vi "MassBandAnalysis.vi"(7 "Settings":T2 {"Bands" items=["No Bands", "", "Test2", "test3", "Test"]; "Smoothing" items=["No smoothing"=0, "1/4 semitone"=25, "1/2 semitone"=50, "1 semitone"=100, "2 semitones"=200]; "View Type" items=["As measured", "Normalize", "Separate", "Complex Average", "Real Average"]}) -> ()   [LabVIEW 2024]
uses:
  ViolinSubs/Mic/Mic_Global.vi
  <vilib>/Analysis/NI_AALBase.lvlib
panel:
  out "Histogram Graph":T1(graph)=[{"X Values"=[17.709212807875016, 17.747951602292737, 17.78669039671046, 17.82542919112818, 17.8641679855459, 17.902906779963622, 17.941645574381344, 17.980384368799065, 18.019123163216786, 18.057861957634508], "Histogram: h(x)"=[2, 0, 0, 0, 0, 0, 1, 1, 0, 1]}, {"X Values"=[12.63540113055175, 12.712222839510153, 12.789044548468555, 12.865866257426957, 12.942687966385359, 13.01950967534376, 13.096331384302163, 13.173153093260565, 13.249974802218967, 13.326796511177369], "Histogram: h(x)"=[1, 0, 0, 1, 1, 0, 0, 1, 0, 1]}, {"X Values"=[19.841497748567125, 19.924216631266706, 20.006935513966287, 20.089654396665868, 20.17237327936545, 20.25509216206503, 20.33781104476461, 20.42052992746419, 20.50324881016377, 20.585967692863353], "Histogram: h(x)"=[1, 0, 1, 0, 0, 0, 0, 1, 0, 2]}, {"X Values"=[13.972825761972334, 14.01058377321214, 14.048341784451946, 14.086099795691752, 14.123857806931557, 14.161615818171363, 14.199373829411169, 14.237131840650974, 14.27488985189078, 14.312647863130586], "Histogram: h(x)"=[1, 0, 1, 1, 0, 0, 0, 1, 0, 1]}]
  in  "intervals":i32=10
  in  "Path":path=path "/Users/crogers/Desktop/Violin/ViolinData/Testing"
  out "# Lines":i32=5
  out "Average FRF":cluster{"x0":dbl, "df":dbl, dbl[]}[](graph)=[{"x0"=0.0, "df"=1.0, array[7000 elements]}, {"x0"=0.0, "df"=1.0, array[7000 elements]}, {"x0"=0.0, "df"=1.0, array[7000 elements]}, {"x0"=0.0, "df"=1.0, array[7000 elements]}, {"x0"=0.0, "df"=1.0, array[7000 elements]}]
  # "1. select the instrument folder (it will get all the TRF files in each test)\n2. hit run\n3. mess with settings (need to do a first run to get the band dropdown \n    to be correct)"
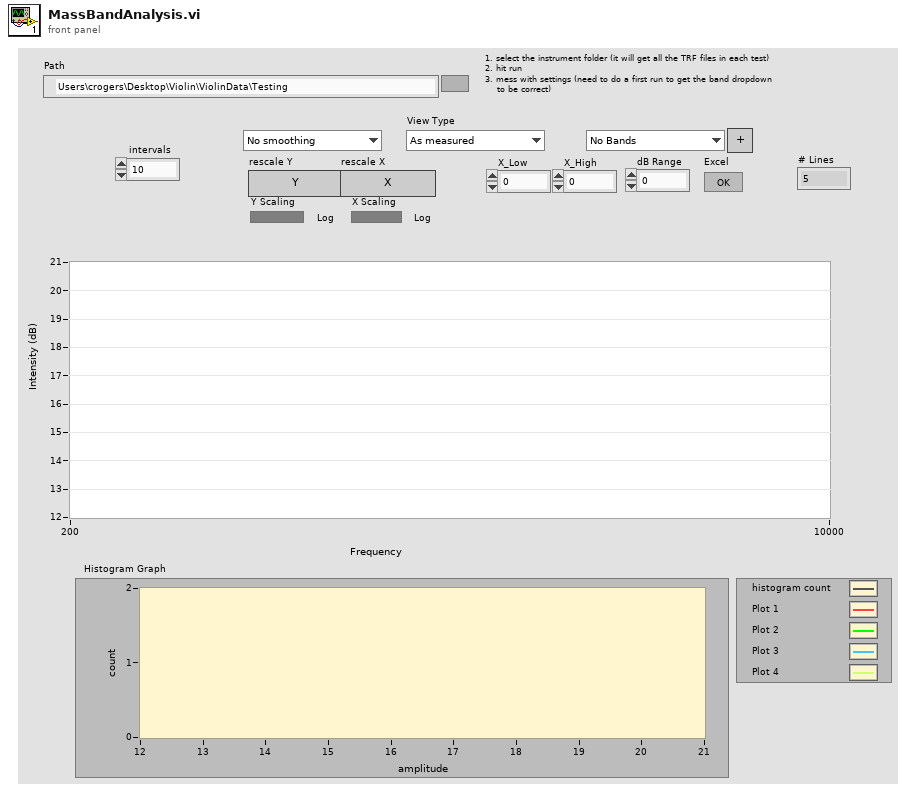
[diagram p1: front panel]
types:
  T1 = cluster{"X Values":dbl[], "Histogram: h(x)":i32[]}[]
  T2 = cluster{"View Type":u16, "Smoothing":u16, "Bands":u16, "New Band":bool, "rescale Y":bool, "rescale X":bool, "X_Low":dbl, "X_High":dbl, "dB Range":dbl, "Excel":bool, "Y Scaling":bool, "X Scaling":bool}
  T3 = cluster{"Start freq":dbl, "Hz resolution":dbl, cdb[]}
  T4 = cluster{"Alerts":bool, "Log X Axis":bool, "dB scale":bool, "Averaging":bool, "Fade":dbl, "Centroids?":bool}
  T5 = cluster{"Band ranges":dbl[][], "CoM":dbl[][], "Band Ave":dbl[][]}
  T6 = cluster{dbl, "df":dbl, "Power Spectrum (V^2 rms)":dbl[]}[]
  T7 = cluster{"X Values":dbl[], "Histogram: h(x)":i32[]}
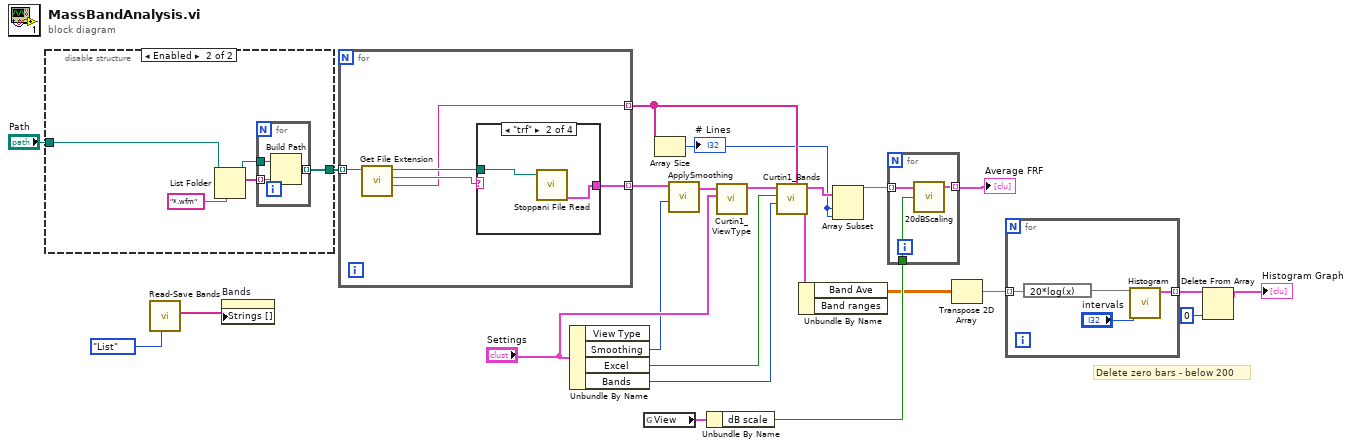
[diagram p0: block diagram]
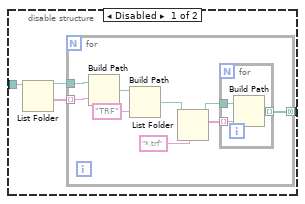
[diagram p2: hidden frame]
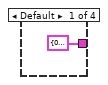
[diagram p3: hidden frame]
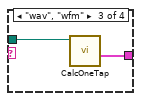
[diagram p4: hidden frame]
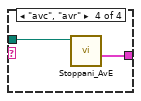
[diagram p5: hidden frame]
diagram:
  # "Delete zero bars - below 200"
  n1 = disable-structure shown="Enabled" {
    disable-tunnel: [w26 w45] -> w14
    disable-tunnel: "Path" -> [w25 w41]
    frame Disabled {
      n2 = List Folder(path=w25) -> (path out=w28:path, folder names=w27:string[])  [unwired: 3 in, 2 out]
      n3 = for {
        tunnel: w28 -> [w37]
        tunnel: w27 -> [w36] mode=indexing
        tunnel: [w30] -> w26 mode=concatenating
        n4 = Build Path(base path=w37, name or relative path=w36) -> (appended path=w29:path)
        n5 = Build Path(base path=w29, name or relative path="TRF") -> (appended path=w34:path)
        n6 = List Folder(path=w34, pattern="*.trf") -> (path out=w32:path, filenames=w31:string[])  [unwired: 2 in, 2 out]
        n7 = for {
          tunnel: w32 -> [w40]
          tunnel: w31 -> [w39] mode=indexing
          tunnel: [w38] -> w30 mode=indexing
          n8 = Build Path(base path=w40, name or relative path=w39) -> (appended path=w38:path)
        }
      }
    }
    frame Enabled {
      n9 = List Folder(path=w41, pattern="*.wfm") -> (path out=w43:path, filenames=w42:string[])  [unwired: 2 in, 2 out]
      n10 = for {
        tunnel: w43 -> [w48]
        tunnel: w42 -> [w47] mode=indexing
        tunnel: [w46] -> w45 mode=indexing
        n11 = Build Path(base path=w48, name or relative path=w47) -> (appended path=w46:path)
      }
    }
  }
  n12 = call "Read-Save Bands.vi"("Task"=enum16{"Save", "Read", "List"}."List") -> ("Long names"=w10:string[])  [unwired: 7 in, 3 out]
  n13 = property on="Bands" class="Ring (strict)"("Strings []"=w10) -> ()  [unwired: 2 in, 2 out]
  n14 = for {
    tunnel: [w53] -> w24 mode=indexing
    tunnel: [w49] -> w15 mode=indexing
    tunnel: w14 -> [w50] mode=indexing
    n15 = call <vilib>:"Get File Extension.vi"("file"=w50) -> ("filename without extension"=w49:string, "lowercase file extension"=w51:string, "dup file"=w52:path)  [unwired: 6 in, 2 out]
    n16 = case shown="\"trf\"" w51 {
      tunnel: [T3 {"Start freq"=0.0, "Hz resolution"=0.0, []} ("Waveform Graph") w55 w57 w60] -> w53
      tunnel: w52 -> [_ w56 w58 w59]
      frame Default {
      }
      frame "trf" {
        n17 = call "Stoppani File Read.vi"("String in"=w56) -> ("Complex FRF"=w55:cluster{"t0":dbl, "dt":dbl, "Y":cdb[]})  [unwired: 2 in, 3 out]
      }
      frame "wav", "wfm" {
        n18 = call "CalcOneTap.vi"("wavform file"=w58) -> ("Complex FRF"=w57:cluster{dbl, "df":dbl, cdb[]})  [unwired: 7 in, 3 out]
      }
      frame "avc", "avr" {
        n19 = call "Stoppani_AvE.vi"("file (use dialog)"=w59) -> ("Complex FRF"=w60:cluster{"t0":dbl, "df":dbl, "Y":cdb[]})  [unwired: 7 in, 3 out]
      }
    }
  }
  n20 = Unbundle By Name("Settings") -> ("Smoothing"=w18:u16, "Excel"=w16:bool, "Bands"=w17:u16)  [unwired: 1 out]
  n21 = global read "Mic_Global.vi" "View"() -> (w21:T4)
  n22 = Array Size(array=w15) -> (size(s)=w12:i32)
  "# Lines" <- w12
  n23 = call "ApplySmoothing.vi"("Smoothing"=w18, "Complex FRF"=w24) -> ("Complex FRF Out"=w23:cluster{dbl, "df":dbl, cdb[]}[])  [unwired: 9 in]
  n24 = Unbundle By Name(w21) -> ("dB scale"=w20:bool)
  n25 = call "Curtin1_ViewType.vi"("Settings"="Settings", "FRF in"=w23) -> ("FRF Out"=w22:cluster{dbl, "df":dbl, dbl[]}[])  [unwired: 8 in, 1 out]
  n26 = call "Curtin1_Bands.vi"("File Names"=w15, "Bands"=w17, "Excel?"=w16, "Magnitude"=w22) -> ("Raw Data"=w8:T5, "Filter"=w13:T6)  [unwired: 6 in]
  n27 = Unbundle By Name(w8) -> ("Band Ave"=w7:dbl[][])  [unwired: 1 out]
  n28 = Array Subset(array=w13, index=w12, length=w12) -> (w6:T6)
  n29 = for {
    tunnel: w20 -> [w63]
    tunnel: w6 -> [w62] mode=indexing
    tunnel: [w61] -> w9 mode=indexing
    n30 = call "20dBScaling.vi"("Average FRF in"=w62, "dB?"=w63) -> ("Average FRF out"=w61:cluster{"x0":dbl, "df":dbl, dbl[]})  [unwired: 4 in, 1 out]
  }
  "Average FRF" <- w9
  n31 = Transpose 2D Array(2D array=w7) -> (transposed array=w2:dbl[][])
  n32 = for {
    tunnel: w2 -> [w65] mode=indexing
    tunnel: [w66] -> w5 mode=indexing
    n33 = expression code="20*log(x)"(w65) -> (w64:dbl[])
    n34 = call <vilib>:"Histogram.vi"("intervals"="intervals", "X"=w64) -> ("Histogram Graph"=w66:T7)  [unwired: 6 in, 3 out]
  }
  n35 = Delete From Array(array=w5, index=0) -> (array with subset deleted=→"Histogram Graph":T1)  [unwired: 1 in, 1 out]
